vi "Write Voltage.vi"(8 "error in":errorcluster, 10 "Voltage":dbl, 11 "6032A in":refnum<class "6032A.lvclass">) -> (0 "error out":errorcluster, 3 "6032A out":refnum<class "6032A.lvclass">)   [LabVIEW 2019, in "6032A.lvlib" / "6032A.lvclass"]
uses:
  Library/6032A.lvclass
  builds/Instruments/PowerSupply.lvlibp/Library/PowerSupply.lvclass
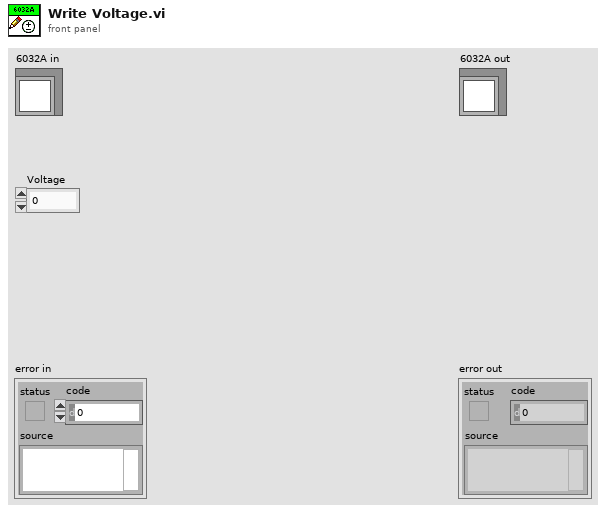
[diagram p1: front panel]
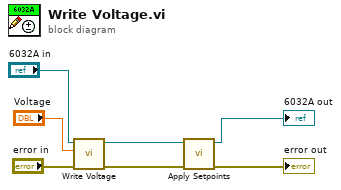
[diagram p0: block diagram]
diagram:
  n1 = call-parent "Write Voltage.vi"("error in"="error in", "Voltage"="Voltage", "PowerSupply in"="6032A in") -> ("error out"=w3:errorcluster, "PowerSupply out"=w4:refnum<class "6032A.lvclass">)  [unwired: 7 in]
  n2 = call "Apply Setpoints.vi"("error in"=w3, "6032A in"=w4) -> ("error out"=→"error out":errorcluster, "6032A out"=→"6032A out":refnum<class "6032A.lvclass">)  [unwired: 8 in]
